vi "Log.vi"(8 "error in (no error)":errorcluster, 9 "Timestamp data points":bool, 10 "tdms file":refnum<k34>, 11 "Start Stream Result in":refnum<class "Start Stream Result.lvclass">) -> (0 "error out":errorcluster, 2 "tdms file out":refnum<k34>, 3 "Start Stream Result out":refnum<class "Start Stream Result.lvclass">)   [LabVIEW 2018, in "Start Stream Result.lvclass"]
uses:
  Start Stream Result.lvclass
  C:/github/NHMFL_Core/Libraries/Instruments/Results/Acquired Result/Acquired Result.lvclass
  Start Stream Result.lvclass/Start Stream Result.ctl
  Acquired Result/Acquired Result.lvclass/Acquired Result.ctl
  Read dt.vi
  Read t0.vi
  Acquired Result/Read Group.vi
  Acquired Result/Read Channels.vi
  Read Scaling coefficients.vi
  Read Configuration.vi
  Acquired Result/Acquired Result.lvclass
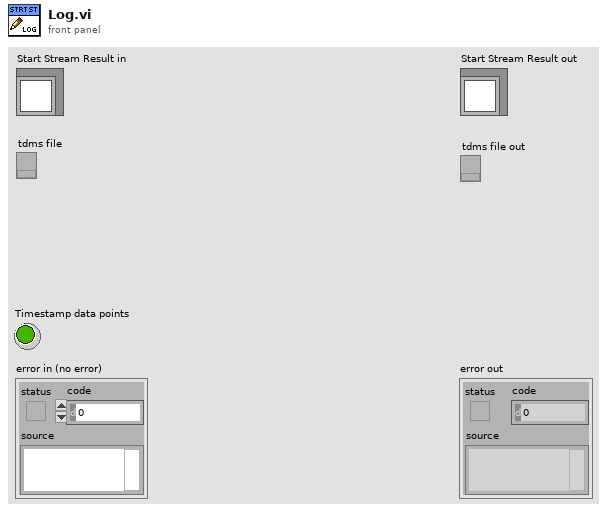
[diagram p1: front panel]
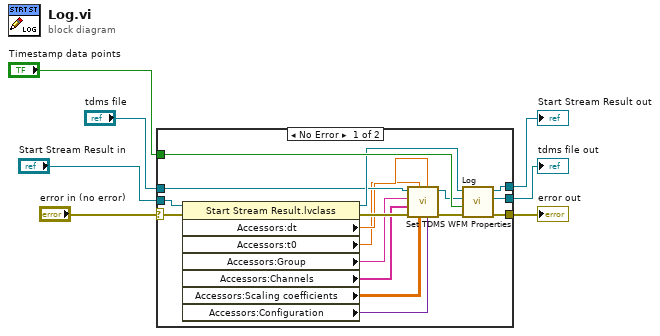
[diagram p0: block diagram]
diagram:
  n1 = case shown="No Error" "error in (no error)" {
    selector: "error in (no error)" -> [w9 w27]
    tunnel: [w24 w27] -> w7
    tunnel: [w23 w26] -> w6
    tunnel: [w22 w25] -> w5
    tunnel: "Timestamp data points" -> [w21 _]
    tunnel: "Start Stream Result in" -> [w18 w25]
    tunnel: "tdms file" -> [w15 w26]
    frame No Error {
      n2 = property class="Start Stream Result.lvclass"(reference=w18, error in=w9) -> (reference out=w17:refnum<class "Start Stream Result.lvclass">, error out=w19:errorcluster, "Accessors:dt"=w12:dbl, "Accessors:t0"=w11:dbl, "Accessors:Group"=w16:string, "Accessors:Channels"=w13:string[], "Accessors:Scaling coefficients"=w10:dbl[][], "Accessors:Configuration"=w8:variant)
      n3 = call "Set TDMS WFM Properties.vi"("Configuration"=w8, "dt"=w12, "Scaling coefficients"=w10, "t0"=w11, "error in (no error)"=w19, "Channel names"=w13, "Group name"=w16, "tdms file"=w15) -> ("error out"=w20:errorcluster, "tdms file out"=w14:refnum<k34>)  [unwired: 2 in]
      n4 = call-parent "Log.vi"("error in (no error)"=w20, "Timestamp data points"=w21, "tdms file"=w14, "Acquired Result in"=w17) -> ("error out"=w24:errorcluster, "tdms file out"=w23:refnum<k34>, "Acquired Result out"=w22:refnum<class "Start Stream Result.lvclass">)  [unwired: 5 in]
    }
    frame Error {
    }
  }
  "error out" <- w7
  "Start Stream Result out" <- w5
  "tdms file out" <- w6
